vi "TestPurePursuit.vi"() -> ()   [LabVIEW 2017]
uses:
  RobotNeededPathData.ctl
panel:
  in  "Max DeAccel":dbl=60.0 format="%#_13g"
  in  "SlowSpeed":dbl=15.0
  in  "SlowDistanceAtEnd":dbl=12.0
  in  "Speed/Curve":dbl=3.0 format="%#_13g"
  in  "Start Location":cluster{dbl, dbl}
  in  "Backwards":bool
  out "Left/Right Power":cluster{"LeftValue":dbl, "RightValue":dbl}(graph)={"LeftValue"=0.4518629712560025, "RightValue"=0.44041361472847607}
  out "Target Vel":dbl(graph)=21.72
  in  "Gains":T1={"FFV"=0.0055, "FFA"=0.0025, "Vel PID"={"P"=0.005, "I"=0.0, "D"=0.0}} {"Vel PID"."D" format="%.5f"; "Vel PID"."I" format="%.3f"; "Vel PID"."P" format="%.3f"}
  out "Graph":cluster{cluster{"x":dbl, "y":dbl}[]}[](graph)=[{[{"x"=0.0, "y"=0.0}, {"x"=5.958901534179709, "y"=-0.041098890268225094}, {"x"=11.913246684108433, "y"=-0.08674605211437728}, {"x"=17.857955768464656, "y"=-0.142022043631154}, {"x"=23.786879154166137, "y"=-0.21308532143857353}, {"x"=29.69212539301894, "y"=-0.307828343937614}, {"x"=35.5631747988101, "y"=-0.4367635370534932}, {"x"=41.385699550923384, "y"=-0.6142118927632001}, {"x"=47.13997273628579, "y"=-0.8598982232374137}, {"x"=52.7986847592069, "y"=-1.2011316327713593}, {"x"=58.323911503765466, "y"=-1.6758323886901672}, {"x"=63.66290542580284, "y"=-2.3367388697970144}, {"x"=68.74221294312689, "y"=-3.2572911759795424}, {"x"=73.45954928168509, "y"=-4.539757346085305}, {"x"=77.67238151068214, "y"=-6.326649219497502}, {"x"=81.18214352358893, "y"=-8.816504015976763}, {"x"=83.71215020112653, "y"=-12.285965429583802}, {"x"=85.54350854077711, "y"=-16.453867196412325}, {"x"=86.87969980341224, "y"=-21.116644757096307}, {"x"=87.86919067185276, "y"=-26.12571575453596}, {"x"=88.62192213320829, "y"=-31.370978987763255}, {"x"=89.22152604993741, "y"=-36.76858013589368}, {"x"=89.73462404390187, "y"=-42.251587769695284}, {"x"=90.21823122952097, "y"=-47.762554690097524}, {"x"=90.72608618767295, "y"=-53.24713964445909}, {"x"=91.31461965757866, "y"=-58.648071685891864}, {"x"=92.04921831034433, "y"=-63.89879327615329}, {"x"=93.01151127961462, "y"=-68.91604392245725}, {"x"=94.30840501928132, "y"=-73.59064420386801}, {"x"=96.08401530311251, "y"=-77.77531118330636}, {"x"=98.53562818808327, "y"=-81.26834553419364}, {"x"=101.9356411323944, "y"=-83.79119920065659}, {"x"=105.99517502353196, "y"=-85.62418265997206}, {"x"=110.49862161662818, "y"=-86.97095723606768}, {"x"=115.27969620765957, "y"=-87.98117310631757}, {"x"=120.20295668007658, "y"=-88.76707264583871}, {"x"=125.1487679129079, "y"=-89.41598209600167}, {"x"=130.0, "y"=-90.0}]}, {[{"x"=72.03556610698088, "y"=-4.510374081701502}, {"x"=83.44069646197207, "y"=-8.241727935955826}]}, {[{"x"=81.18214352358893, "y"=-8.816504015976763}]}, {[{"x"=82.03556610698088, "y"=-4.510374081701502}, {"x"=81.81704211431894, "y"=-2.431257173523909}, {"x"=81.1710206834069, "y"=-0.4430076509435006}, {"x"=80.12573605073035, "y"=1.3674784412232297}, {"x"=78.72687217056946, "y"=2.921074173072439}, {"x"=77.03556610698088, "y"=4.149879956142883}, {"x"=75.12573605073035, "y"=5.0001910812500325}, {"x"=73.08085073965742, "y"=5.434844871981231}, {"x"=70.99028147430435, "y"=5.434844871981231}, {"x"=68.94539616323141, "y"=5.000191081250034}, {"x"=67.03556610698088, "y"=4.149879956142885}, {"x"=65.3442600433923, "y"=2.9210741730724425}, {"x"=63.94539616323141, "y"=1.3674784412232306}, {"x"=62.900111530554874, "y"=-0.4430076509434979}, {"x"=62.25409009964282, "y"=-2.431257173523905}, {"x"=62.03556610698088, "y"=-4.510374081701501}, {"x"=62.25409009964282, "y"=-6.589490989879093}, {"x"=62.90011153055487, "y"=-8.5777405124595}, {"x"=63.94539616323141, "y"=-10.388226604626233}, {"x"=65.3442600433923, "y"=-11.941822336475443}, {"x"=67.03556610698088, "y"=-13.170628119545885}, {"x"=68.94539616323141, "y"=-14.020939244653036}, {"x"=70.99028147430434, "y"=-14.455593035384236}, {"x"=73.08085073965741, "y"=-14.455593035384236}, {"x"=75.12573605073035, "y"=-14.02093924465304}, {"x"=77.03556610698087, "y"=-13.170628119545892}, {"x"=78.72687217056946, "y"=-11.941822336475447}, {"x"=80.12573605073035, "y"=-10.388226604626237}, {"x"=81.17102068340688, "y"=-8.577740512459512}, {"x"=81.81704211431894, "y"=-6.589490989879101}, {"x"=82.03556610698088, "y"=-4.510374081701505}]}, {[{"x"=99.62925706965552, "y"=-42.57097515925139}, {"x"=98.75416094168116, "y"=-34.24499166522433}, {"x"=96.16711845772768, "y"=-26.282893602387723}, {"x"=91.98119578835099, "y"=-19.032662862472954}, {"x"=86.37933784048836, "y"=-12.81116931928134}, {"x"=79.60637268715818, "y"=-7.890322094688614}, {"x"=71.95831140585365, "y"=-4.485185825254277}, {"x"=63.76941097403755, "y"=-2.7445813056092874}, {"x"=55.39756563528416, "y"=-2.7445813056092803}, {"x"=47.208665203468044, "y"=-4.485185825254277}, {"x"=39.56060392216352, "y"=-7.890322094688614}, {"x"=32.78763876883335, "y"=-12.811169319281326}, {"x"=27.185780820970706, "y"=-19.03266286247295}, {"x"=22.99985815159402, "y"=-26.282893602387713}, {"x"=20.41281566764053, "y"=-34.24499166522432}, {"x"=19.53771953966617, "y"=-42.57097515925138}, {"x"=20.41281566764053, "y"=-50.89695865327843}, {"x"=22.999858151594005, "y"=-58.85905671611504}, {"x"=27.1857808209707, "y"=-66.10928745602982}, {"x"=32.787638768833325, "y"=-72.33078099922143}, {"x"=39.560603922163494, "y"=-77.25162822381415}, {"x"=47.20866520346804, "y"=-80.6567644932485}, {"x"=55.397565635284124, "y"=-82.39736901289349}, {"x"=63.76941097403752, "y"=-82.3973690128935}, {"x"=71.95831140585365, "y"=-80.6567644932485}, {"x"=79.60637268715816, "y"=-77.25162822381418}, {"x"=86.37933784048835, "y"=-72.33078099922146}, {"x"=91.98119578835099, "y"=-66.10928745602983}, {"x"=96.16711845772767, "y"=-58.85905671611509}, {"x"=98.75416094168116, "y"=-50.89695865327847}, {"x"=99.62925706965552, "y"=-42.5709751592514}]}]
  in  "Max Accel":dbl=120.0 format="%#_13g"
  in  "MaxVel":dbl(slide)=71.32867132867133 scale=0.0..150.0
  in  "LookAhead":dbl=10.0
  in  "Path":cluster{"x":dbl, "y":dbl}[](array[cluster])=[{"x"=0.0, "y"=0.0}, {"x"=90.0, "y"=0.0}, {"x"=90.0, "y"=-90.0}, {"x"=130.0, "y"=-90.0}]
  in  "Config":T2={"Gear Reduction"=8.7, "Wheel Radius (m)"=0.076, "# Motors"=3, "coeff of friction"=0.1, "Mass (kg)"=55.0, "Motor"={"Ke (V)"=0.0183, "R (ohms)"=0.14, "KT (Nm/A)"=0.0183, "Tf (Nm)"=0.015}}
  # ".007"
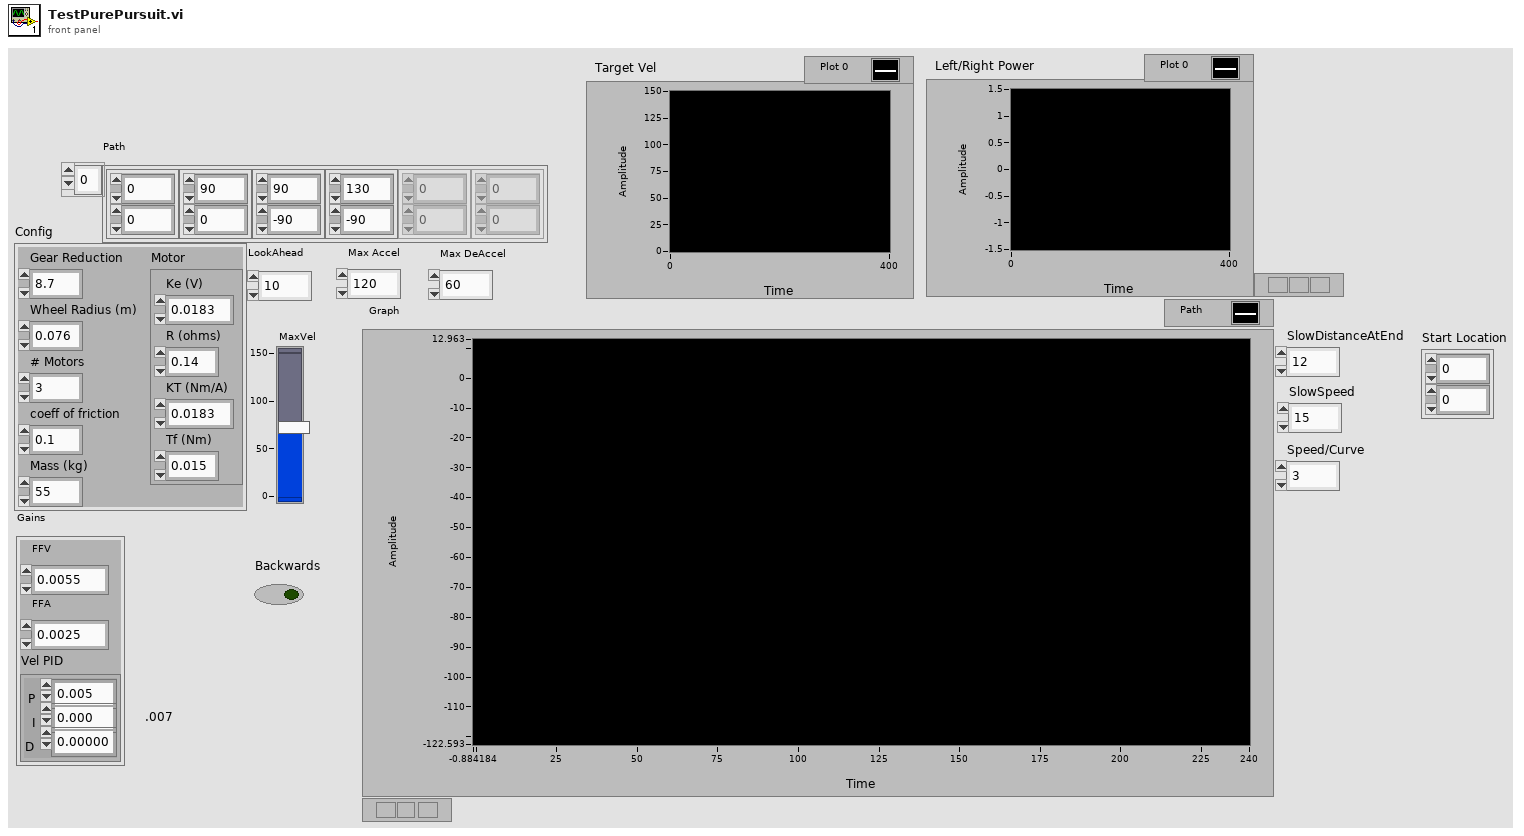
[diagram p1: front panel]
types:
  T1 = cluster{"FFV":dbl, "FFA":dbl, "Vel PID":cluster{"P":dbl, "I":dbl, "D":dbl}}
  T2 = cluster{"Gear Reduction":dbl, "Wheel Radius (m)":dbl, "# Motors":u32, "coeff of friction":dbl, "Mass (kg)":dbl, "Motor":cluster{"Ke (V)":dbl, "R (ohms)":dbl, "KT (Nm/A)":dbl, "Tf (Nm)":dbl}}
  T3 = typedef "RobotNeededPathData.ctl" = cluster{"Path":cluster{dbl, dbl}[], "MaxVel":dbl, "MaxAccel":dbl, "Backwards?":bool, "PointSpacing":dbl, "LookaheadDist":dbl, "Speed/Curve":dbl, "SlowDistanceAtEnd":dbl, "SlowSpeed":dbl, "MaxDeAccel":dbl}
  T4 = cluster{"Left Distance":dbl, "Right Distance":dbl, "dx/dt":dbl, "dx/dt":dbl, dbl, "Location":cluster{dbl, dbl}}
  T5 = cluster{"Left Distance":dbl, "Right Distance":dbl, "dx/dt":dbl, "dx/dt":dbl, dbl, cluster{dbl, dbl}}
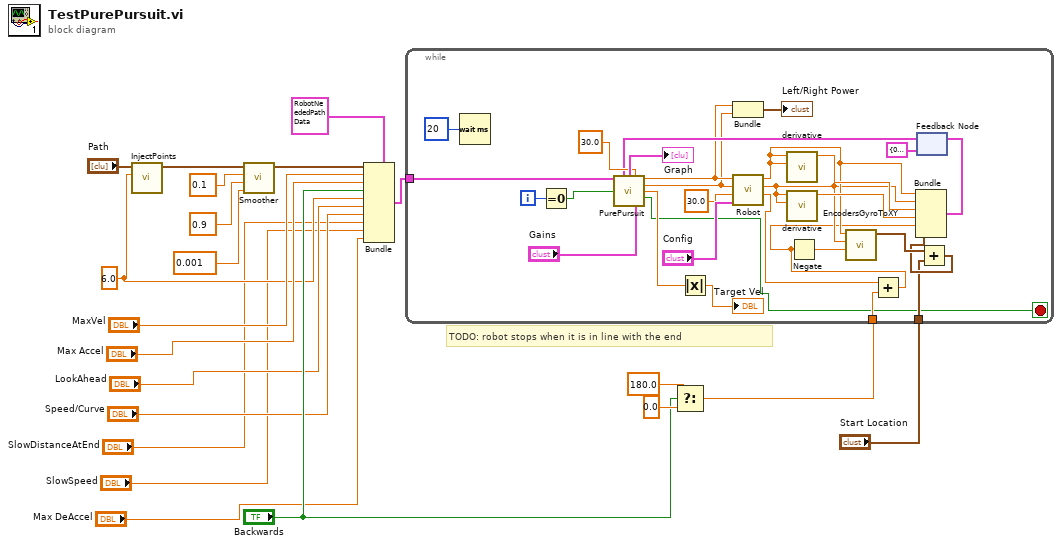
[diagram p0: block diagram]
diagram:
  w6 = 6.0 ("Distance")
  # "TODO: robot stops when it is in line with the end"
  n1 = call "InjectPoints.vi"("Spacing"=w6, "Path"="Path") -> ("Path out"=w16:cluster{dbl, dbl}[])  [unwired: 9 in]
  n2 = call "Smoother.vi"("tolerance"=0.001, "B"=0.9, "A"=0.1, "Path"=w16) -> ("SmoothPath"=w15:cluster{dbl, dbl}[])  [unwired: 7 in]
  n3 = Bundle(cluster=T3 {"Path"=[], "MaxVel"=0.0, "MaxAccel"=0.0, "Backwards?"=FALSE, "PointSpacing"=0.0, "LookaheadDist"=0.0, "Speed/Curve"=1.8, "SlowDistanceAtEnd"=12.0, "SlowSpeed"=15.0, "MaxDeAccel"=0.0} ("RobotNeededPathData"), "Path"=w15, "MaxVel"="MaxVel", "MaxAccel"="Max Accel", "Backwards?"="Backwards", "PointSpacing"=w6, "LookaheadDist"="LookAhead", "Speed/Curve"="Speed/Curve", "SlowDistanceAtEnd"="SlowDistanceAtEnd", "SlowSpeed"="SlowSpeed", "MaxDeAccel"="Max DeAccel") -> (w17:T3)
  n4 = Select(t=180.0, s="Backwards", f=0.0) -> (s? t:f=w12:dbl)
  n5 = while {
    tunnel: w17 -> [w25]
    tunnel: w12 -> [w31]
    tunnel: "Start Location" -> [w26]
    i -> [w37]
    stop <- w22 stop-if-true
    n6 = Wait (ms)(milliseconds to wait=u32 20) -> ()  [unwired: 1 out]
    n7 = Equal To 0?(x=w37) -> (x = 0?=w36:bool)
    n8 = feedback #1(T4 {"Left Distance"=0.0, "Right Distance"=0.0, "dx/dt"=0.0, "dx/dt"=0.0, 0.0, "Location"={0.0, 0.0}}) -> (w39:T4)
    n9 = call "PurePursuit.vi"("RobotNeededPathData"=w25, "SensorData"=w39, "Trackwidth"=30.0, "Reset"=w36, "Gains"="Gains") -> ("Graph"=→"Graph":cluster{cluster{"x":dbl, "y":dbl}[]}[], "LeftValue"=w35:dbl, "RightValue"=w34:dbl, "TargetVel"=w24:dbl, "Done"=w22:bool)  [unwired: 6 in]
    n10 = Absolute Value(x=w24) -> (abs(x)=→"Target Vel":dbl)
    n11 = Bundle("LeftValue"=w35, "RightValue"=w34) -> (→"Left/Right Power":cluster{"LeftValue":dbl, "RightValue":dbl})  [unwired: 1 in]
    n12 = call "Robot.vi"("Config"="Config", "WheelBase"=30.0, "Right Value"=w34, "Left Value"=w35) -> ("Angle"=w32:dbl, "Right Distance"=w38:dbl, "Left Distance"=w41:dbl)  [unwired: 5 in]
    n13 = call "derivative.vi"("Starting value"=w41, "x"=w41) -> ("dx/dt"=w43:dbl)  [unwired: 9 in]
    n14 = call "derivative.vi"("Starting value"=w38, "x"=w38) -> ("dx/dt"=w42:dbl)  [unwired: 9 in]
    n15 = Add(x=w32, y=w31) -> (x+y=w30:dbl)
    n16 = Negate(x=w30) -> (-x=w40:dbl)
    n17 = call "EncodersGyroToXY.vi"("Angle (degrees)"=w40, "Right Distance"=w38, "Left Distance"=w41) -> ("Location"=w28:cluster{dbl, dbl})  [unwired: 8 in]
    n18 = Add(x=w28, y=w26) -> (x+y=w27:cluster{dbl, dbl})
    n19 = Bundle("Left Distance"=w41, "Right Distance"=w38, "dx/dt"=w43, "dx/dt"=w42, w30, w27) -> (w47:T5)  [unwired: 1 in]
    n20 = feedback-in #1(w47) -> ()
  }
